vi "Generate Error for Combo Box not found.vi"(0 "Template combox path":path, 11 "error in (no error)":errorcluster) -> (15 "error out":errorcluster)   [LabVIEW 2021, in "Migrator.lvlib"]
uses:
  Migrator.lvlib
  <vilib>/ErrorRing/Error Ring.xnode
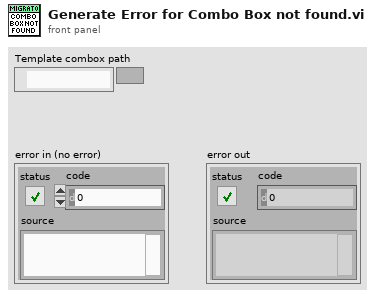
[diagram p1: front panel]
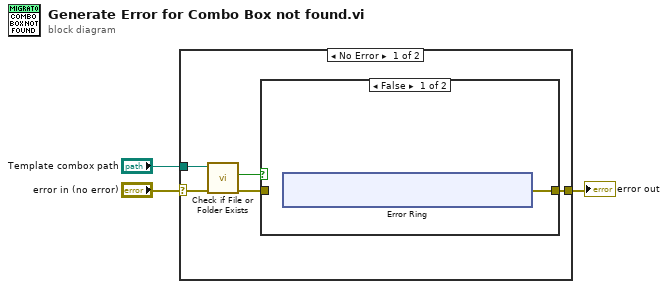
[diagram p0: block diagram]
diagram:
  n1 = case shown="No Error" "error in (no error)" {
    selector: "error in (no error)" -> [w5 w12]
    tunnel: [w8 w12] -> w3
    tunnel: "Template combox path" -> [w4 _]
    frame No Error {
      n2 = call <vilib>:"Check if File or Folder Exists.vi"("error in (no error)"=w5, "path"=w4) -> ("error out"=w7:errorcluster, "file or folder exists?"=w6:bool)  [unwired: 7 in, 1 out]
      n3 = case shown="False" w6 {
        tunnel: w7 -> [_ w11]
        tunnel: [w9 w11] -> w8
        frame False {
          n4 = xnode "Error Ring"() -> ("error out"=w9:errorcluster)
        }
        frame True {
        }
      }
    }
    frame Error {
    }
  }
  "error out" <- w3
